vi "Update Controls.vi"(8 "error in":errorcluster, 10 "MHL References":T2, 11 "MHL Status":T1) -> (0 "error out":errorcluster)   [LabVIEW 2020]
uses:
  controls/MHL References.ctl
  TrioMotion Controller/Connection Type.ctl
  controls/MHL Status.ctl
  TrioMotion Controller/TrioMotion Controller.lvlib
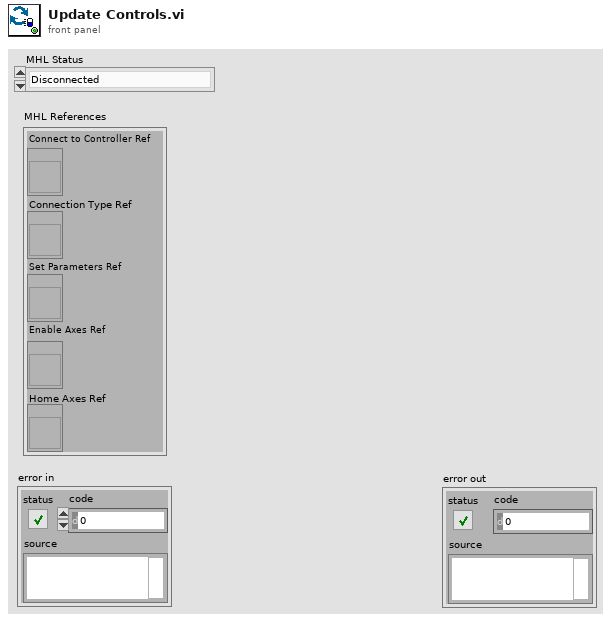
[diagram p1: front panel]
types:
  T1 = typedef "MHL Status.ctl" = enum16{"Disconnected", "Connecting", "Connected", "Axes Enabled", "Machine Running", "Shutdown"}
  T2 = typedef "MHL References.ctl" = cluster{"Connect to Controller Ref":refnum<vi>, "Connection Type Ref":refnum<vi>, "Set Parameters Ref":refnum<vi>, "Enable Axes Ref":refnum<vi>, "Home Axes Ref":refnum<vi>}
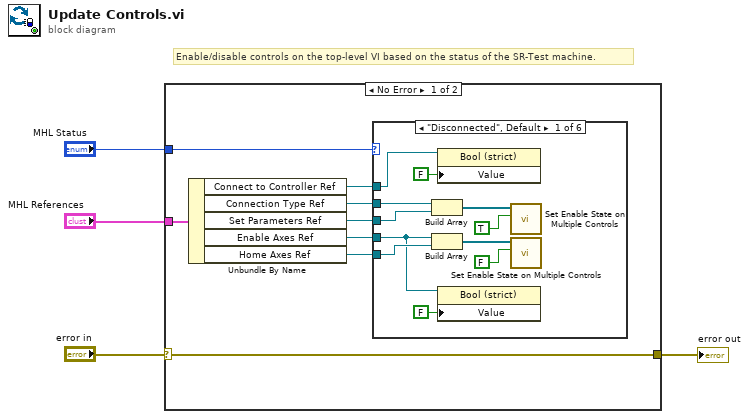
[diagram p0: block diagram]
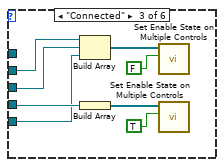
[diagram p3: hidden frame]
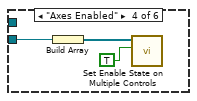
[diagram p4: hidden frame]
diagram:
  # "Enable/disable controls on the top-level VI based on the status of the SR-Test machine."
  n1 = case shown="No Error" "error in" {
    selector: "error in" -> [w12 w35]
    tunnel: [w12 w35] -> w3
    tunnel: "MHL Status" -> [w11 _]
    tunnel: "MHL References" -> [w10 _]
    frame No Error {
      n2 = Unbundle By Name(w10) -> ("Connect to Controller Ref"=w9:refnum<vi>, "Connection Type Ref"=w8:refnum<vi>, "Set Parameters Ref"=w7:refnum<vi>, "Enable Axes Ref"=w6:refnum<vi>, "Home Axes Ref"=w5:refnum<vi>)
      n3 = case shown="\"Disconnected\", Default" w11 {
        tunnel: w9 -> [w16 _ _ _ _ _]
        tunnel: w8 -> [w19 _ w25 _ _ _]
        tunnel: w7 -> [w18 _ w26 _ _ _]
        tunnel: w6 -> [w14 _ w27 _ _ _]
        tunnel: w5 -> [w17 _ w24 w32 _ _]
        frame "Disconnected", Default {
          n4 = Build Array(w19, w18) -> (w21:refnum<vi>[])
          n5 = Build Array(w14, w17) -> (w22:refnum<vi>[])
          n6 = property class="Bool (strict)"(reference=w16, "Value"=FALSE) -> ()  [unwired: 1 in, 2 out]
          n7 = property class="Bool (strict)"(reference=w14, "Value"=FALSE) -> ()  [unwired: 1 in, 2 out]
          n8 = call "Set Enable State on Multiple Controls.vi"("Enable?"=TRUE, "Controls"=w21) -> ()  [unwired: 10 in]
          n9 = call "Set Enable State on Multiple Controls.vi"("Enable?"=FALSE, "Controls"=w22) -> ()  [unwired: 10 in]
        }
        frame "Connecting" {
        }
        frame "Connected" {
          n10 = Build Array(w25, w26, w24) -> (w29:refnum<vi>[])
          n11 = Build Array(w27) -> (w30:refnum<vi>[])
          n12 = call "Set Enable State on Multiple Controls.vi"("Enable?"=FALSE, "Controls"=w29) -> ()  [unwired: 10 in]
          n13 = call "Set Enable State on Multiple Controls.vi"("Enable?"=TRUE, "Controls"=w30) -> ()  [unwired: 10 in]
        }
        frame "Axes Enabled" {
          n14 = Build Array(w32) -> (w33:refnum<vi>[])
          n15 = call "Set Enable State on Multiple Controls.vi"("Enable?"=TRUE, "Controls"=w33) -> ()  [unwired: 10 in]
        }
        frame "Machine Running" {
        }
        frame "Shutdown" {
        }
      }
    }
    frame Error {
    }
  }
  "error out" <- w3
